vi "Ctor from Config.vi"(6 "Platforms":refnum<class "PlatformManager.lvclass">, 7 "Resource":refnum<class "Resource.lvclass">, 8 "error in (no error)":errorcluster, 9 "Version":string, 10 "Alias":string, 11 "Device Key":T1) -> (0 "error out":errorcluster, 3 "Device out":refnum<class "Device.lvclass">)   [LabVIEW 2020, in "PicoG-App.lvlib" / "Device.lvclass"]
uses:
  Device.lvclass
  Device Key.ctl
  Builds/picoG/ppl/PicoG-Core.lvlibp/PicoG-Processor/PicoG-Core/Resource/Resource.lvclass
  Builds/picoG/ppl/PicoG-Core.lvlibp/PicoG-Processor/PicoG-Core/PlatformManager/PlatformManager.lvclass
  Ref Data.ctl
  Resource Ref.ctl
  Device.lvclass/Device.ctl
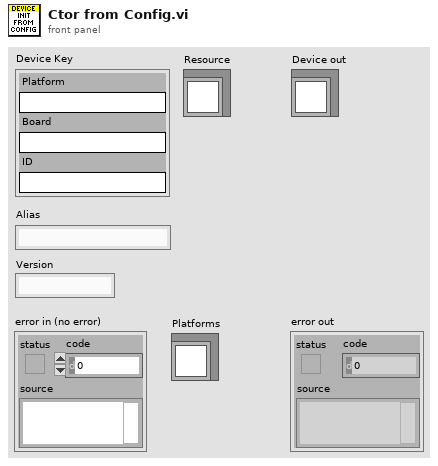
[diagram p1: front panel]
types:
  T1 = typedef "PicoG-App.lvlib/Device.lvclass/Device Key.ctl" = cluster{"Platform":string, "Board":string, "ID":string}
  T2 = typedef "PicoG-App.lvlib/Device.lvclass/Resource Ref.ctl" = cluster{"Resource":refnum<class "Resource.lvclass">, "Open":bool, "At Prompt":bool, "Running":bool}
  T3 = typedef "PicoG-App.lvlib/Device.lvclass/Ref Data.ctl" = cluster{"Alias":string, "Version":string, "Build":timestamp, "Key":T1}
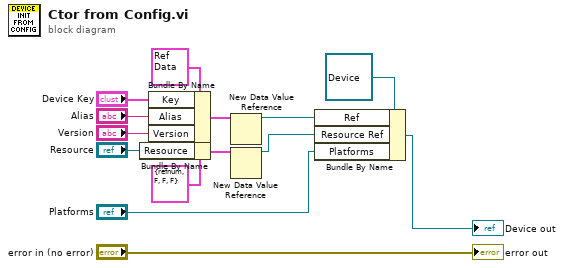
[diagram p0: block diagram]
diagram:
  n1 = Bundle By Name(cluster=T2 {"Resource"=refnum, "Open"=FALSE, "At Prompt"=FALSE, "Running"=FALSE} ("Resource Ref"), "Resource"="Resource") -> (w6:T2)
  n2 = Bundle By Name(cluster=T3 {"Alias"="", "Version"="", "Build"=timestamp(0 s since 1904-01-01), "Key"={"Platform"="", "Board"="", "ID"=""}} ("Ref Data"), "Key"="Device Key", "Alias"="Alias", "Version"="Version") -> (w9:T3)
  n3 = New Data Value Reference(data value=w9) -> (data value reference=w4:refnum<data-value>)  [unwired: 1 in, 1 out]
  n4 = New Data Value Reference(data value=w6) -> (data value reference=w3:refnum<data-value>)  [unwired: 1 in, 1 out]
  n5 = Bundle By Name(cluster=refnum<class "Device.lvclass"> refnum ("Device in"), "Ref"=w4, "Resource Ref"=w3, "Platforms"="Platforms") -> (→"Device out":refnum<class "Device.lvclass">)
  "error out" <- "error in (no error)"
